vi "mqttCmdInitialize.vi"(8 "error in (no error)":errorcluster, 11 "mqttCmd in":refnum<class "mqttCmd.lvclass">) -> (0 "error out":errorcluster, 3 "mqttCmd out":refnum<class "mqttCmd.lvclass">)   [LabVIEW 2020, in "mqttCmd.lvclass"]
uses:
  mqttCmd.lvclass
  mqtt.lvclass
panel:
  in  "mqtt instance":refnum<class "mqtt.lvclass">
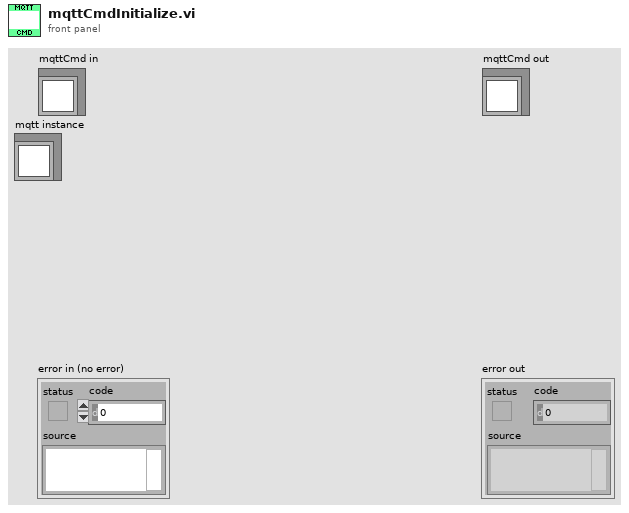
[diagram p1: front panel]
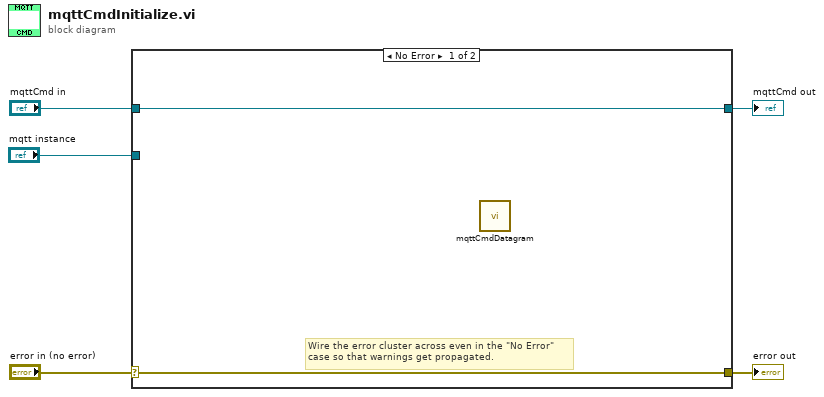
[diagram p0: block diagram]
diagram:
  n1 = case shown="No Error" "error in (no error)" {
    selector: "error in (no error)" -> [w6 w9]
    tunnel: [w6 w9] -> w4
    tunnel: [w7 w8] -> w2
    tunnel: "mqttCmd in" -> [w7 w8]
    tunnel: "mqtt instance" -> [_ _]
    frame No Error {
      # "Wire the error cluster across even in the \"No Error\"\ncase so that warnings get propagated."
      n2 = call "mqttCmdDatagram.vi"() -> ()  [unwired: 9 in, 3 out]
    }
    frame Error {
    }
  }
  "error out" <- w4
  "mqttCmd out" <- w2
